vi "TcpServer.vi"(10 "Port in (0)":u16, 11 "IpAddress (127.0.0.1)":string="127.0.0.1") -> (0 "error out":errorcluster, 2 "Log":string, 3 "Port out":u16)   [LabVIEW 2021]
uses:
  TcpServer/TcpServer/TcpServer.lvclass
  TcpServer/Connection/Connection.lvclass
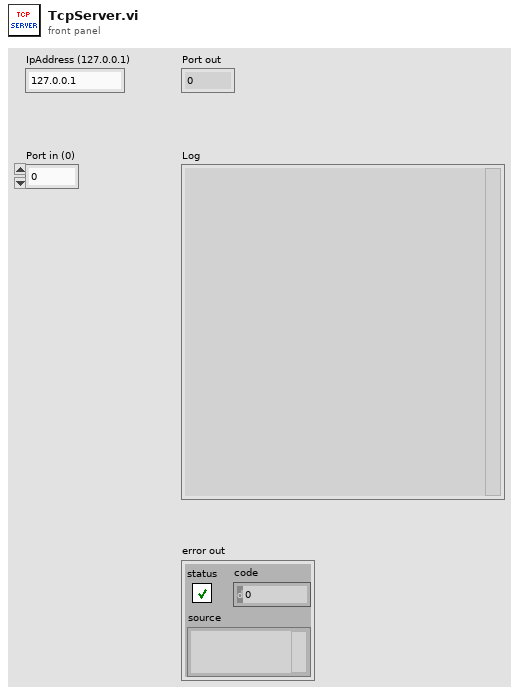
[diagram p1: front panel]
types:
  T1 = enum16{"Standard", "Buffered", "CRLF", "Immediate"}
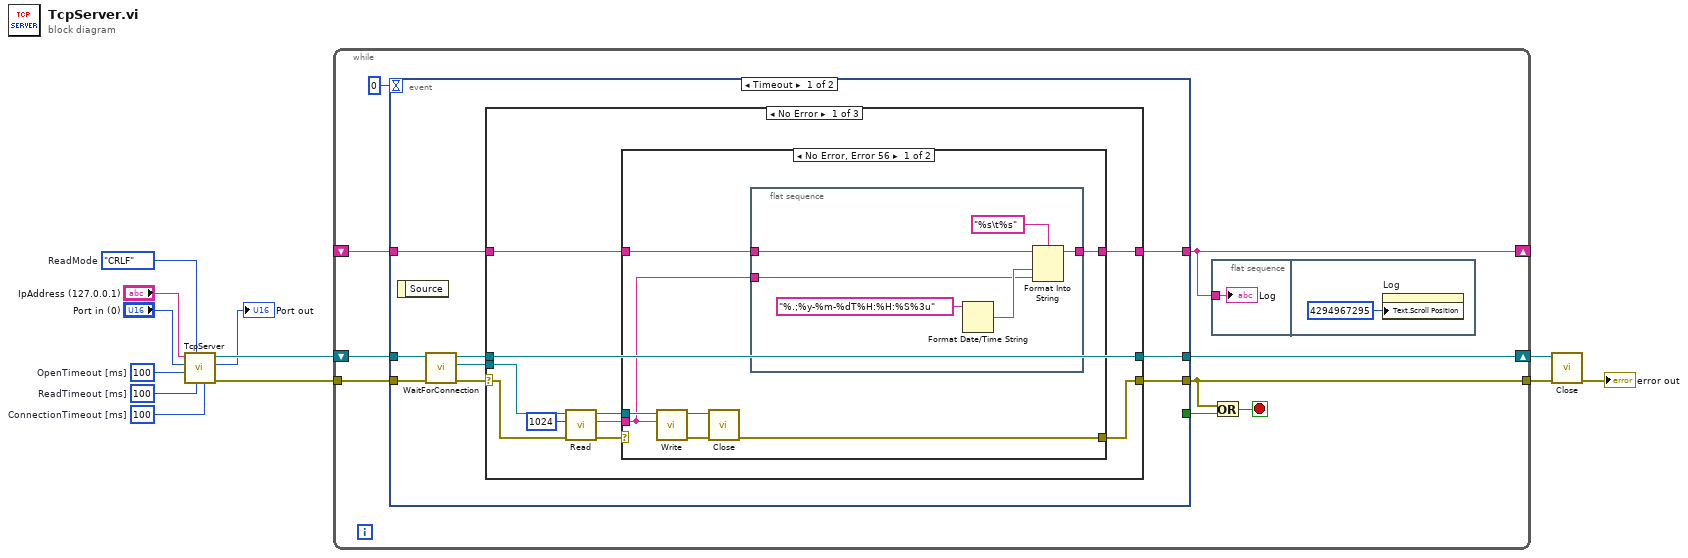
[diagram p0: block diagram]
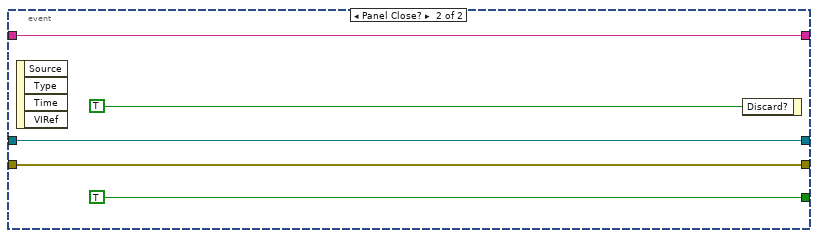
[diagram p5: hidden frame]
diagram:
  w1 = 100  # ReadTimeout [ms]
  w5 = 100  # OpenTimeout [ms]
  w2 = 100  # ConnectionTimeout [ms]
  w6 = T1."CRLF"  # ReadMode
  n1 = call "TcpServer.vi"("ConnectionTimeout [ms] (5000)"=w2, "ReadTimeout [ms] (5000)"=w1, "ReadMode (Standard)"=w6, "OpenTimeout [ms] (5000)"=w5, "Port in (0)"="Port in (0)", "IpAddress (127.0.0.1)"="IpAddress (127.0.0.1)") -> ("error out"=w10:errorcluster, "Port out"=→"Port out":u16, "TcpServer"=w4:refnum<class "TcpServer.lvclass">)  [unwired: 3 in]
  n2 = while {
    tunnel: w10 -> [w21]
    shift-right: [w19] -> w7
    shift-left: w4 -> [w20]
    tunnel: [w16] -> w9
    shift-right: [w13] -> _
    shift-left: _ -> [w14]
    stop <- w17 stop-if-true
    n3 = event shown="[0] Timeout" {
      selector: _ -> [_ _]
      dyn-events: _ -> [_ _]
      timeout: 0 -> [_ _]
      tunnel: w21 -> [w32 w66]
      tunnel: w20 -> [w31 w67]
      tunnel: [w28 w67] -> w19
      tunnel: [w26 w66] -> w16
      tunnel: [_ TRUE] -> w18
      tunnel: w14 -> [w25 w63]
      tunnel: [w24 w63] -> w13
      event Timeout {
        n4 = event-data() -> ()  [unwired: 1 in, 1 out]
        n5 = call-dynamic "WaitForConnection.vi"("error in (no error)"=w32, "TcpServer in"=w31) -> ("error out"=w29:errorcluster, "Connection"=w30:refnum<class "Connection.lvclass">, "TcpServer out"=w27:refnum<class "TcpServer.lvclass">)  [unwired: 7 in]
        n6 = case shown="No Error" w29 {
          selector: w29 -> [w38 w59 _]
          tunnel: w30 -> [w40 _ _]
          tunnel: [w42 w60 w62] -> w28
          tunnel: w27 -> [w42 w60 w62]
          tunnel: [w41 w59 _] -> w26
          tunnel: w25 -> [w33 w58 w61]
          tunnel: [w34 w58 w61] -> w24
          frame No Error {
            n7 = call-dynamic "Read.vi"("error in (no error)"=w38, "BytesToRead"=1024, "Connection in"=w40) -> ("error out"=w35:errorcluster, "Data"=w37:string, "Connection out"=w39:refnum<class "Connection.lvclass">)  [unwired: 6 in]
            n8 = case shown="No Error, Error 56" w35 {
              selector: w35 -> [_ w57]
              tunnel: [w47 w57] -> w41
              tunnel: w39 -> [w46 _]
              tunnel: w37 -> [w45 _]
              tunnel: [w44 w56] -> w34
              tunnel: w33 -> [w43 w56]
              frame No Error {
                n9 = call-dynamic "Write.vi"("Data"=w45, "Connection in"=w46) -> ("error out"=w48:errorcluster, "Connection out"=w49:refnum<class "Connection.lvclass">)  [unwired: 8 in]
                n10 = call-dynamic "Close.vi"("error in (no error)"=w48, "Connection"=w49) -> ("error out"=w47:errorcluster)  [unwired: 9 in]
                n11 = flat-sequence {
                  tunnel: w45 -> [w52]
                  tunnel: [w51] -> w44
                  tunnel: w43 -> [w50]
                  frame #0 {
                    n12 = Format Date/Time String(time format string (%c)="%.;%y-%m-%dT%H:%H:%S%3u") -> (date/time string=w55:string)  [unwired: 2 in]
                    n13 = Format Into String(format string="%s\t%s", initial string=w50, w55, w52) -> (resulting string=w51:string)  [unwired: 1 in, 1 out]
                  }
                }
              }
              frame Default {
              }
            }
          }
          frame Default {
          }
          frame Error {
            # "Timeout"
          }
        }
      }
      event Panel Close? {
        n14 = event-data() -> ()  [unwired: 1 in, 4 out]
        n15 = event-data("Discard?"=TRUE) -> ()  [unwired: 1 in, 1 out]
      }
    }
    n16 = flat-sequence {
      tunnel: w13 -> [w22]
      frame #0 {
        "Log" <- w22
      }
      frame #1 {
        n17 = property on="Log" class="Str"("Text.Scroll Position"=u32 4294967295) -> ()  [unwired: 2 in, 2 out]
      }
    }
    n18 = Or(x=w16, y=w18) -> (x .or. y?=w17:bool)
  }
  n19 = call-dynamic "Close.vi"("error in (no error)"=w9, "TcpSocket in"=w7) -> ("error out"=→"error out":errorcluster)  [unwired: 8 in, 1 out]
